vi "PWR SUPP IOLINK.vi"(5 "OCP":bool, 7 "OVP":bool, 8 "ON/OFF":bool, 9 "Voltage in":dbl=24.0 min=0.0 max=30.1 step=0.1 format="%#_g V", 10 "Current in":dbl=1.0 min=0.0 max=5.0 step=0.001 format="%#_4g A", 11 "VISA in":refnum<visa-resource-name>="COM2") -> (2 "Curent [A]":dbl(knob) scale=0.0..5.0 scale format="%#_3g", 3 "Voltage":dbl(knob) scale=0.0..30.0, 4 "error out":errorcluster)   [LabVIEW 2022 SP3]
panel:
  # "Power supply on / off"
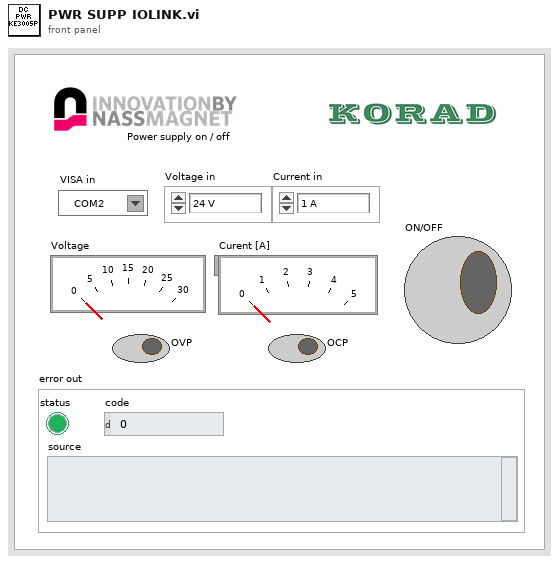
[diagram p1: front panel]
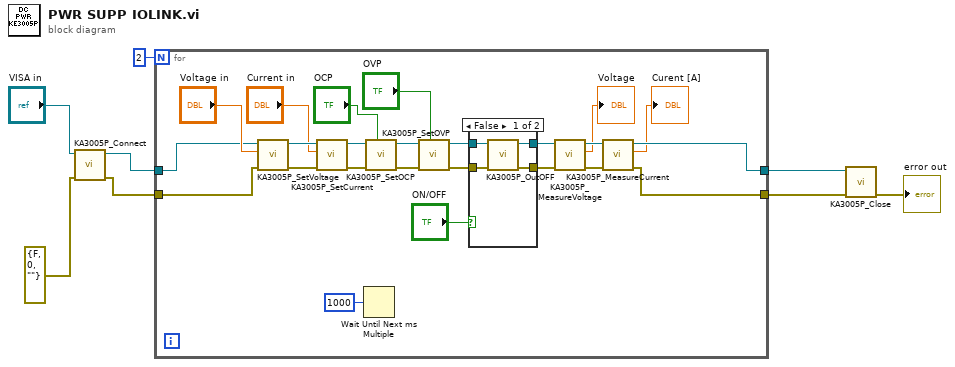
[diagram p0: block diagram]
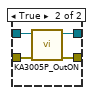
[diagram p2: hidden frame]
diagram:
  n1 = call <vilib>:"KA3005P_Connect.vi"("error in (no error)"=errorcluster {"status"=FALSE, "code"=0, "source"=""}, "VISA resource name in"="VISA in") -> ("error out"=w6:errorcluster, "VISA resource name out"=w7:refnum<visa-resource-name>)  [unwired: 8 in]
  n2 = for {
    N: 2 -> [_]
    tunnel: w7 -> [w28]
    tunnel: [w19] -> w3
    tunnel: w6 -> [w27]
    tunnel: [w20] -> w4
    n3 = call <vilib>:"KA3005P_SetVoltage.vi"("error in (no error)"=w27, "Voltage in"="Voltage in", "VISA resource name in"=w28) -> ("error out"=w26:errorcluster, "VISA resource name out"=w31:refnum<visa-resource-name>)  [unwired: 7 in]
    n4 = call <vilib>:"KA3005P_SetCurrent.vi"("error in (no error)"=w26, "Current in"="Current in", "VISA resource name in"=w31) -> ("error out"=w11:errorcluster, "VISA resource name out"=w12:refnum<visa-resource-name>)  [unwired: 7 in]
    n5 = Wait Until Next ms Multiple(millisecond multiple=u32 1000) -> ()  [unwired: 1 out]
    n6 = call <vilib>:"KA3005P_SetOCP.vi"("ON (F)"="OCP", "error in (no error)"=w11, "VISA resource name in"=w12) -> ("error out"=w14:errorcluster, "VISA resource name out"=w13:refnum<visa-resource-name>)  [unwired: 7 in]
    n7 = call <vilib>:"KA3005P_SetOVP.vi"("ON (F)"="OVP", "error in (no error)"=w14, "VISA resource name in"=w13) -> ("error out"=w16:errorcluster, "VISA resource name out"=w15:refnum<visa-resource-name>)  [unwired: 7 in]
    n8 = case shown="False" "ON/OFF" {
      tunnel: w15 -> [w36 w40]
      tunnel: w16 -> [w35 w39]
      tunnel: [w33 w38] -> w24
      tunnel: [w34 w37] -> w23
      frame False {
        n9 = call <vilib>:"KA3005P_OutOFF.vi"("error in (no error)"=w35, "VISA resource name in"=w36) -> ("error out"=w34:errorcluster, "VISA resource name out"=w33:refnum<visa-resource-name>)  [unwired: 8 in]
      }
      frame True {
        n10 = call <vilib>:"KA3005P_OutON.vi"("error in (no error)"=w39, "VISA resource name in"=w40) -> ("error out"=w37:errorcluster, "VISA resource name out"=w38:refnum<visa-resource-name>)  [unwired: 8 in]
      }
    }
    n11 = call <vilib>:"KA3005P_MeasureVoltage.vi"("error in (no error)"=w23, "VISA resource name in"=w24) -> ("error out"=w21:errorcluster, "Voltage"=→"Voltage":dbl, "VISA resource name out"=w22:refnum<visa-resource-name>)  [unwired: 7 in]
    n12 = call <vilib>:"KA3005P_MeasureCurrent.vi"("error in (no error)"=w21, "VISA resource name in"=w22) -> ("error out"=w20:errorcluster, "Curent [A]"=→"Curent [A]":dbl, "VISA resource name out"=w19:refnum<visa-resource-name>)  [unwired: 7 in]
  }
  n13 = call <vilib>:"KA3005P_Close.vi"("error in (no error)"=w4, "VISA resource name in"=w3) -> ("error out"=→"error out":errorcluster)  [unwired: 9 in]
